vi "config PIGEON2.vi"(8 "error in (no error)":errorcluster) -> (0 "error out":errorcluster)   [LabVIEW 2023]
uses:
  Global INIT.vi
  <vilib>/Rock Robotics/WPI/ThirdParty/Phoenix-LabVIEW/Pigeon2/CTRE_Phoenix_Pigeon2_GetFaults.vi
  <vilib>/Rock Robotics/WPI/ThirdParty/Phoenix-LabVIEW/Pigeon2/CTRE_Phoenix_Pigeon2_GetStickyFaults.vi
  <vilib>/Rock Robotics/WPI/ThirdParty/Phoenix-LabVIEW/Pigeon2/controls/CTRE_Phoenix_Pigeon2_Configurables.ctl
  <vilib>/Rock Robotics/WPI/ThirdParty/Phoenix-LabVIEW/Pigeon2/controls/CTRE_Phoenix_Pigeon2_Faults.ctl
panel:
  out "Sticky Faults":T1
  out "Faults":T1
  out "Configurables":T2
  # "Yaw Angle needed to reach the current orientation in degrees"
  # "Configures the mounting pose of the Pigeon2\nThis is the yaw-pitch-roll teh Pigeon2 underwent to get to its current orientation,\n referenced from the robot's point of view\nThis is only necessary if the Pigeon2 is mounted at an exotic angle near the gimbal lock point or not forward.\nIf the pigeon is relatively flat and pointed forward, this is not needed"
  # "Pitch Angle needed to reach the current orientation in degrees"
  # "Roll Angle needed to reach the current orientation in degrees"
  # "Disables the temperature compensation\nfrom the Pigeon2. It is recommended that\nthis remains false"
  # "Disables the no-motion calibration from the\nPigeon2. It is recommended that this \nremains false"
  # "Enables the compass for Pigeon2\nThis is not recommended for any indoor robotics"
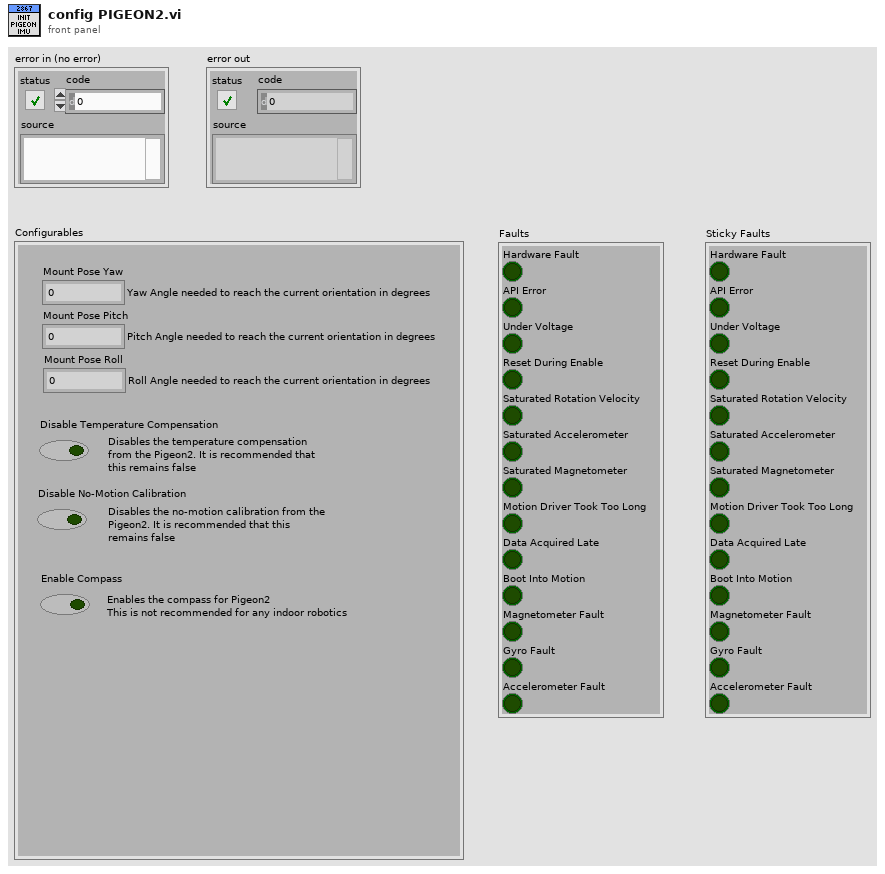
[diagram p1: front panel]
types:
  T1 = typedef "CTRE_Phoenix_Pigeon2_Faults.ctl" = cluster{"Hardware Fault":bool, "API Error":bool, "Under Voltage":bool, "Reset During Enable":bool, "Saturated Rotation Velocity":bool, "Saturated Accelerometer":bool, "Saturated Magnetometer":bool, "Motion Driver Took Too Long":bool, "Data Acquired Late":bool, "Boot Into Motion":bool, "Magnetometer Fault":bool, "Gyro Fault":bool, "Accelerometer Fault":bool}
  T2 = typedef "CTRE_Phoenix_Pigeon2_Configurables.ctl" = cluster{"Mount Pose Yaw":dbl, "Mount Pose Pitch":dbl, "Mount Pose Roll":dbl, "Disable Temperature Compensation":bool, "Disable No-Motion Calibration":bool, "Enable Compass":bool}
  T3 = typedef "ctrl ctre pigeon2 config.ctl" = cluster{"Installed?":bool, "Configurables":T2, "CAN ID":u8, "refnum name":string, "CAN bus":string}
  T4 = typedef "CTRE_PigeonIMU_DeviceRef.ctl" = cluster{"DeviceStatus":errorcluster, "Device Number":u8, "Type":T5, "Device ID":u32, "Handle":u64, "UsageFrame":u32, "Library Path":path}
  T5 = typedef "CTRE_PigeonIMU_ConnectionType.ctl" = u32
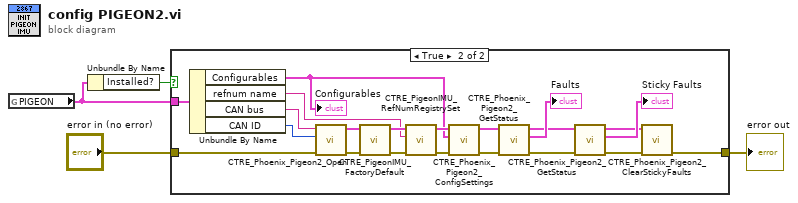
[diagram p0: block diagram]
diagram:
  n1 = global read "Global INIT.vi" "PIGEON"() -> (w2:T3)
  n2 = Unbundle By Name(w2) -> ("Installed?"=w3:bool)
  n3 = case shown="True" w3 {
    tunnel: "error in (no error)" -> [w5 w26]
    tunnel: w2 -> [_ w18]
    tunnel: [w5 w8] -> w1
    frame False {
    }
    frame True {
      n4 = Unbundle By Name(w18) -> ("Configurables"=w15:T2, "refnum name"=w16:string, "CAN bus"=w17:string, "CAN ID"=w19:u8)
      "Configurables" <- w15
      n5 = call <vilib>:"CTRE_Phoenix_Pigeon2_Open.vi"("error in"=w26, "Device Number"=w19, "canbus"=w17) -> ("error out"=w25:errorcluster, "PigeonIMUDevRef"=w24:T4)  [unwired: 7 in]
      n6 = call <vilib>:"CTRE_PigeonIMU_FactoryDefault.vi"("error in"=w25, "PigeonIMUDevRef"=w24) -> ("error out"=w23:errorcluster, "PigeonIMUDevRef"=w22:T4)  [unwired: 8 in]
      n7 = call <vilib>:"CTRE_PigeonIMU_RefNumRegistrySet.vi"("error in (no error)"=w23, "refnum name"=w16, "PigeonIMUDevRef"=w22) -> ("error out"=w21:errorcluster, "PigeonIMUDevRef"=w20:T4)  [unwired: 7 in]
      n8 = call <vilib>:"CTRE_Phoenix_Pigeon2_ConfigSettings.vi"("error in (no error)"=w21, "Pigeon2 Configurables"=w15, "PigeonIMUDevRef 2"=w20) -> ("error out"=w13:errorcluster, "PigeonIMUDevRef"=w14:T4)  [unwired: 7 in]
      n9 = call-poly <vilib>:"CTRE_Phoenix_Pigeon2_GetStatus.vi"("error in"=w13, "Pigeon2DevRef"=w14) -> ("error out"=w6:errorcluster, "Faults"=→"Faults":T1, "Pigeon2DevRef"=w7:T4)  [unwired: 7 in]
      n10 = call-poly <vilib>:"CTRE_Phoenix_Pigeon2_GetStatus.vi"("error in"=w6, "Pigeon2DevRef 2"=w7) -> ("error out"=w10:errorcluster, "Faults"=→"Sticky Faults":T1, "Pigeon2DevRef"=w9:T4)  [unwired: 7 in]
      n11 = call <vilib>:"CTRE_Phoenix_Pigeon2_ClearStickyFaults.vi"("error in"=w10, "PigeonIMUDevRef 2"=w9) -> ("error out"=w8:errorcluster)  [unwired: 8 in, 1 out]
    }
  }
  "error out" <- w1
